vi "Data Replay Run Test.vi"() -> ()   [LabVIEW 2015]
uses:
  Data File Loader/AngleReference.ctl
  IP Source/Analog Replay/Load Input.ctl
  IP Source/Analog Replay/Settings.ctl
  IP Source/Analog Replay/Input.ctl
  IP Source/APU/Input.ctl
  <vilib>/rvi/interface/RandomDataEmulation/nirviRandomDataOpen.vi
  <vilib>/rvi/interface/common/niFpgaCacheSessionInfoDynamic.vi
  <vilib>/Utility/error.llb/Error Cluster From Error Code.vi
  <vilib>/rvi/errors/niLvFpgaAdjustHostInterfaceError.vi
  <vilib>/FPGAPlugInAG/Dynamic/niLvFpga_Run_Dynamic.vi
  <vilib>/FPGAPlugInAG/Dynamic/niLvFpga_Close_Dynamic.vi
  <vilib>/rvi/interface/nirviOpenFPGA/nirviOpenFPGA.xnode
  Compile Tests/APU + 1 Data Replay.vi
  <vilib>/rvi/interface/nirviReadWriteControl/nirviReadWriteControl.xnode
  <vilib>/rvi/interface/nirviMethod/nirviMethod.xnode
  <vilib>/rvi/interface/nirviCloseFPGA/nirviCloseFPGA.xnode
  <vilib>/rvi/interface/Simulation/niFpgaSimulationCallBeginRW.vi
  IP Source/Analog Replay/Analog Replay.lvlib
  IP Source/APU/APU.lvlib
  NiFpgaLv.dll
panel:
  in  "max AO voltage value":dbl
  in  "memory size":i32=32768
  out "Load done":bool
  out "Load time (s)":dbl=9.013101180287777
  in  "Offset":dbl format="%#_15g"
  in  "Reverse Negate":bool
  in  "RPM":dbl=500.0 format="%#_15g"
  in  "stop":bool
  in  "threshold speed (RPM)":dbl
  in  "threshold voltage":dbl
  in  "maximum speed (RPM)":dbl=10000.0
  in  "maximum voltage":dbl=10.0
  out "Data":dbl[](graph)
  out "Selected Offset":i32=2705
  out "Selected Length":i32=3178
  in  "CycleAngle?":T1
  in  "ReverseData":bool
  in  "MissingTeeth Location":dbl=200.0
  in  "File Path":path=path "C:/Users/sbarrett/Documents/SVN/Engine Simulation/Engine Sim FPGA Example/crank VR data.csv"
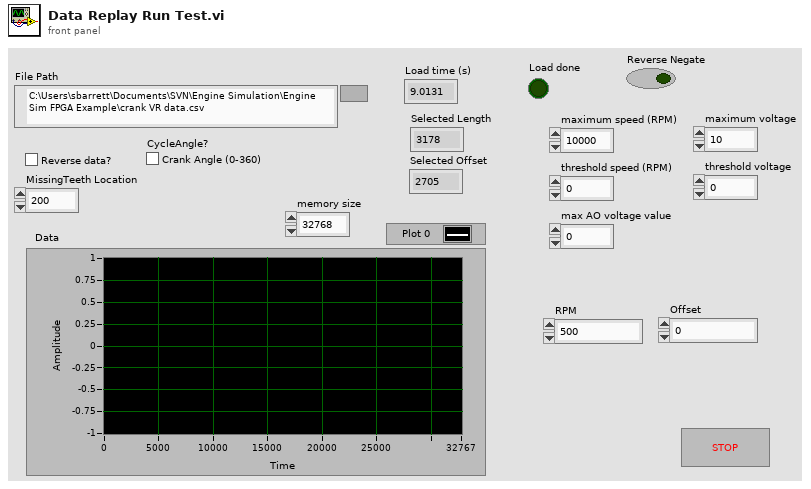
[diagram p1: front panel]
types:
  T1 = typedef "AngleReference.ctl" = bool
  T2 = typedef "Engine Simulation Toolkit.lvlib/Analog Replay.lvlib/Settings.ctl" = cluster{"ReverseNegate":bool, "CycleAngle":bool, "SpeedThreshold":fxp<+/-,23,2>, "AOBelowThreshold":i16}
  T3 = typedef "Engine Simulation Toolkit.lvlib/Analog Replay.lvlib/Load Input.ctl" = cluster{"Data":i16[], "LoadOffset":u16, "Done":bool}
  T4 = typedef "Engine Simulation Toolkit.lvlib/APU.lvlib/Input.ctl" = cluster{"desired speed":fxp<+/-,23,2>, "reset":bool}
  T5 = typedef "Engine Simulation Toolkit.lvlib/Analog Replay.lvlib/Input.ctl" = cluster{"Offset":i16, "VScaleSlope":fxp<+,18,6>, "VScaleIntercept":fxp<+/-,18,3>}
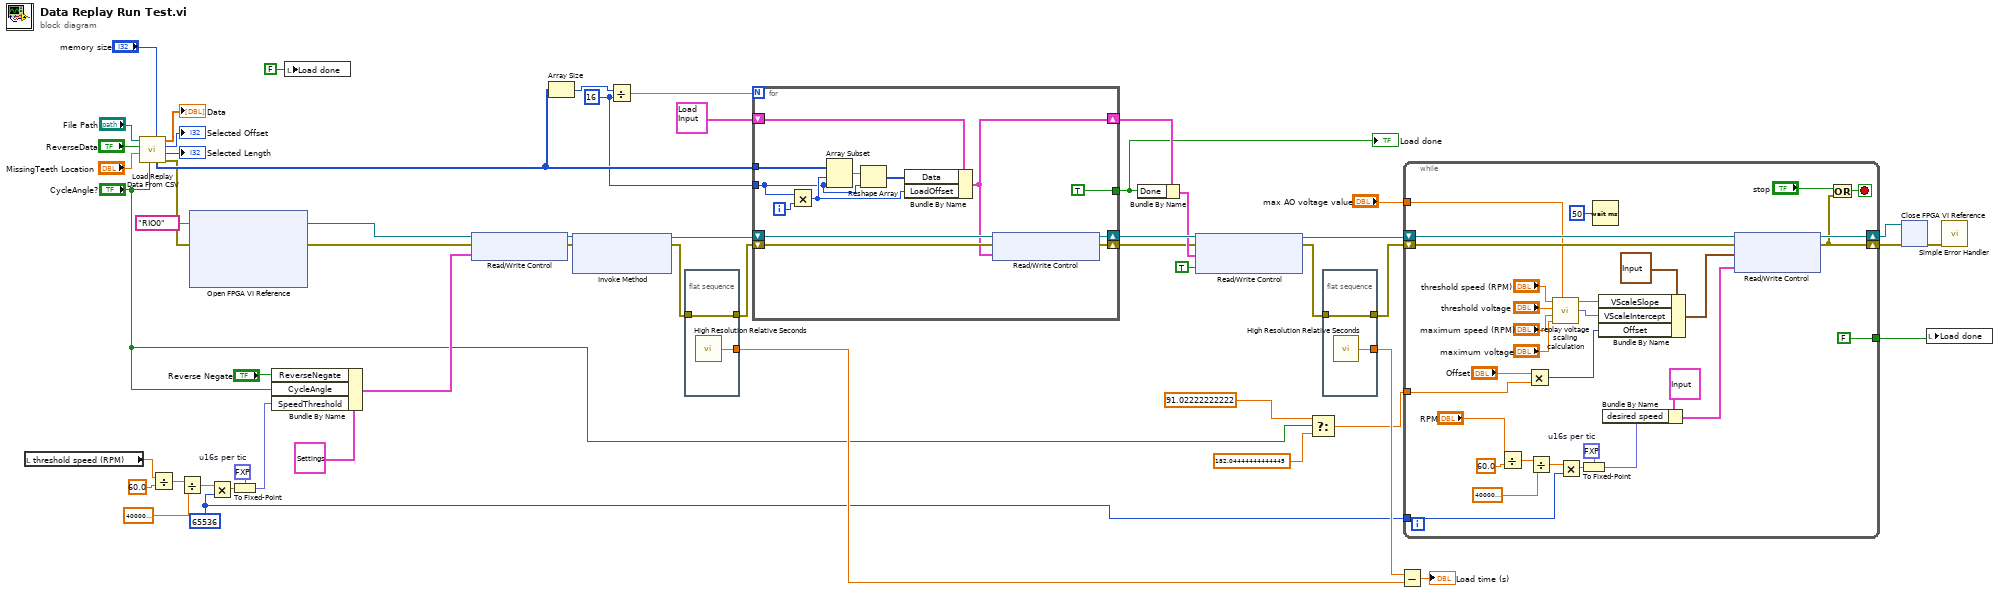
[diagram p0: block diagram]
diagram:
  w12 = fxp<+/-,23,2> 0.0  # u16s per tic
  w10 = u32 65536 ("n")
  w27 = 16 ("y")
  n1 = local read "threshold speed (RPM)"() -> (w4:dbl)
  n2 = call "Load Replay Data From CSV.vi"("Memory Size as number"="memory size", "CycleAngle?"="CycleAngle?", "MissingTeeth Location"="MissingTeeth Location", "ReverseData"="ReverseData", "File Path"="File Path") -> ("error out"=w41:errorcluster, "Selected Length"=→"Selected Length":i32, "Selected Offset"=→"Selected Offset":i32, "Data"=→"Data":dbl[], "DAC data"=w55:i16[])  [unwired: 2 in]
  n3 = Divide(x=w4, y=60.0) -> (x/y=w16:dbl)
  n4 = Divide(x=w16, y=40000000.0) -> (x/y=w13:dbl)
  n5 = xnode "Open FPGA VI Reference"("error in"=w41, "resource name"=tag "RIO0") -> ("FPGA VI Reference Out"=w24:refnum<k20>, "error out"=w51:errorcluster)
  n6 = Multiply(x=w13, y=w10) -> (x*y=w11:dbl)
  n7 = To Fixed-Point(fixed-point type=w12, number=w11) -> (fixed-point=w5:fxp<+/-,23,2>)
  n8 = Bundle By Name(cluster=T2 {"ReverseNegate"=FALSE, "CycleAngle"=FALSE, "SpeedThreshold"=0.0, "AOBelowThreshold"=0} ("analog data replay settings v1.0.0"), "ReverseNegate"="Reverse Negate", "CycleAngle"="CycleAngle?", "SpeedThreshold"=w5) -> (w50:T2)
  n9 = local write "Load done"(FALSE ("Load done")) -> ()
  n10 = xnode "Read/Write Control"("FPGA VI Reference In"=w24, "error in"=w51, "settings.my replay"=w50) -> ("FPGA VI Reference Out"=w36:refnum<k20>, "error out"=w22:errorcluster)
  n11 = Array Size(array=w55) -> (size(s)=w37:i32)
  n12 = xnode "Invoke Method"("FPGA VI Reference In"=w36, "error in"=w22) -> ("FPGA VI Reference Out"=w35:refnum<k20>, "error out"=w33:errorcluster)  [unwired: 1 in]
  n13 = Divide(x=w37, y=w27) -> (x/y=w38:dbl)
  n14 = flat-sequence {
    tunnel: [w57] -> w34
    tunnel: w33 -> [w57]
    tunnel: [w56] -> w31
    frame #0 {
      n15 = call <vilib>:"High Resolution Relative Seconds.vi"() -> ("relative seconds"=w56:dbl)
    }
  }
  n16 = for {
    N: w38 -> [_]
    shift-right: [w64] -> w19
    shift-left: w34 -> [w67]
    tunnel: w55 -> [w70]
    tunnel: w27 -> [w58]
    shift-right: [w65] -> w29
    shift-left: w35 -> [w66]
    shift-right: [w60] -> w26
    shift-left: T3 {"Data"=[0, 0, 0, 0, 0, 0, 0, 0, 0, 0, 0, 0, 0, 0, 0, 0], "LoadOffset"=0, "Done"=FALSE} ("my replay") -> [w63]
    tunnel: [TRUE ("Done")] -> w23
    i -> [w68]
    n17 = Multiply(x=w58, y=w68) -> (x*y=w59:i32)
    n18 = Array Subset(array=w70, index=w59, length=w58) -> (w69:i16[])
    n19 = Reshape Array(w69, w58) -> (w62:i16[])
    n20 = Bundle By Name(cluster=w63, "Data"=w62, "LoadOffset"=w59) -> (w60:T3)
    n21 = xnode "Read/Write Control"("FPGA VI Reference In"=w66, "error in"=w67, "load input.my replay"=w60) -> ("FPGA VI Reference Out"=w65:refnum<k20>, "error out"=w64:errorcluster)
  }
  "Load done" <- w23
  n22 = Bundle By Name(cluster=w26, "Done"=w23) -> (w25:T3)
  n23 = xnode "Read/Write Control"("FPGA VI Reference In"=w29, "error in"=w19, "load input.my replay"=w25, "go.my apu"=TRUE) -> ("FPGA VI Reference Out"=w28:refnum<k20>, "error out"=w18:errorcluster)
  n24 = Select(t=91.02222222222 ("y"), s="CycleAngle?", f=182.04444444444445 ("y")) -> (s? t:f=w6:dbl)
  n25 = flat-sequence {
    tunnel: [w72] -> w17
    tunnel: w18 -> [w72]
    tunnel: [w71] -> w32
    frame #0 {
      n26 = call <vilib>:"High Resolution Relative Seconds.vi"() -> ("relative seconds"=w71:dbl)
    }
  }
  n27 = Subtract(x=w32, y=w31) -> (x-y=→"Load time (s)":dbl)
  n28 = while {
    shift-right: [w94] -> w54
    shift-left: w17 -> [w103]
    shift-right: [w97] -> w53
    shift-left: w28 -> [w102]
    tunnel: [FALSE ("Load")] -> w40
    tunnel: w10 -> [w76]
    tunnel: w6 -> [w74]
    tunnel: "max AO voltage value" -> [w73]
    stop <- w95 stop-if-true
    w79 = fxp<+/-,23,2> 0.0  # u16s per tic
    n29 = Divide(x="RPM", y=60.0) -> (x/y=w83:dbl)
    n30 = Multiply(x="Offset", y=w74) -> (x*y=w84:i16)
    n31 = Divide(x=w83, y=40000000.0) -> (x/y=w80:dbl)
    n32 = call "replay voltage scaling calculation.vi"("max ao voltage"=w73, "maximum voltage"="maximum voltage", "maximum speed (RPM)"="maximum speed (RPM)", "threshold voltage"="threshold voltage", "threshold speed (RPM)"="threshold speed (RPM)") -> ("intercept (b)"=w90:fxp<+/-,18,3>, "slope (m)"=w91:fxp<+,18,6>)  [unwired: 5 in]
    n33 = Multiply(x=w80, y=w76) -> (x*y=w78:dbl)
    n34 = To Fixed-Point(fixed-point type=w79, number=w78) -> (fixed-point=w75:fxp<+/-,23,2>)
    n35 = Wait (ms)(milliseconds to wait=u32 50) -> ()  [unwired: 1 out]
    n36 = Bundle By Name(cluster=T5 {"Offset"=0, "VScaleSlope"=0.0, "VScaleIntercept"=0.0} ("my replay"), "VScaleSlope"=w91, "VScaleIntercept"=w90, "Offset"=w84) -> (w89:T5)
    n37 = Bundle By Name(cluster=T4 {"desired speed"=0.0, "reset"=FALSE} ("my apu"), "desired speed"=w75) -> (w87:T4)
    n38 = xnode "Read/Write Control"("FPGA VI Reference In"=w102, "error in"=w103, "input.my replay"=w89, "input.my apu"=w87) -> ("FPGA VI Reference Out"=w97:refnum<k20>, "error out"=w94:errorcluster)
    n39 = Or(x="stop", y=w94) -> (x .or. y?=w95:bool)
  }
  n40 = xnode "Close FPGA VI Reference"("FPGA VI Reference In"=w53, "error in"=w54) -> ("error out"=w52:errorcluster)
  n41 = local write "Load done"(w40) -> ()
  n42 = call <vilib>:"Simple Error Handler.vi"("error in (no error)"=w52) -> ()  [unwired: 4 in, 5 out]
